vi "FlpLib DQtoABC_noSine_PowInv 4.vi"(0 "direct":sgl format="%#_30g", 1 "cosx":sgl, 2 "sinx":sgl, 5 "quadrature":sgl format="%#_30g") -> (4 "A":sgl format="%#_32g", 6 "B":sgl, 8 "C":sgl, 10 "alpha":sgl format="%#_30g", 15 "beta":sgl format="%#_30g")   [LabVIEW 2017]
uses:
  DQtoAlphaBeta_noSine/FlpLib DQtoAlphaBeta_noSine 4.vi
  AlphaBetaToABC_PowInv/FlpLib AlphaBetaToABC_PowInv 4.vi
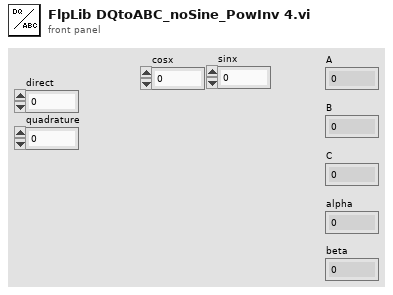
[diagram p1: front panel]
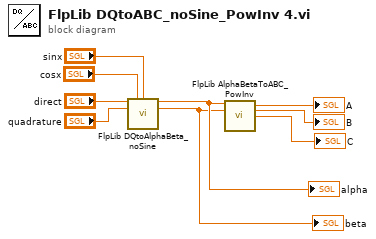
[diagram p0: block diagram]
diagram:
  n1 = call-poly "FlpLib DQtoAlphaBeta_noSine.vi"("direct"="direct", "cosx"="cosx", "sinx"="sinx", "quadrature"="quadrature") -> ("alpha"=w6:sgl, "beta"=w5:sgl)  [unwired: 10 in]
  "alpha" <- w6
  "beta" <- w5
  n2 = call-poly "FlpLib AlphaBetaToABC_PowInv.vi"("alpha"=w6, "beta"=w5) -> ("A"=→"A":sgl, "B"=→"B":sgl, "C"=→"C":sgl)  [unwired: 11 in]
